vi "Parse Elements Treewise.vi"(4 "VI Data in":T1[](array[typedef]), 5 "XPath Get Attribute":T5[](array[typedef]), 6 "Parents":string[](array[string]), 7 "XPath Node Attribute":T5, 8 "error in":errorcluster, 9 "Attribute":string[](array[string]), 10 "XML File Path":path, 11 "Node in":refnum<k20>) -> (0 "error out":errorcluster, 2 "VI Data out":T1[](array[typedef]), 3 "Node out":refnum<k20>)   [LabVIEW 2020, in "VI Properties Editor.lvlib"]
uses:
  VI Properties Editor.lvlib
  <vilib>/xml/NI_XML.lvlib
  <vilib>/xml/Close Reference(Node).vi
  CTLs/XPath Get Attribute.ctl
  <vilib>/picture/picture.llb/imagedata.ctl
  CTLs/VI Properties.ctl
  CTLs/Control Properties.ctl
  CTLs/VI Data.ctl
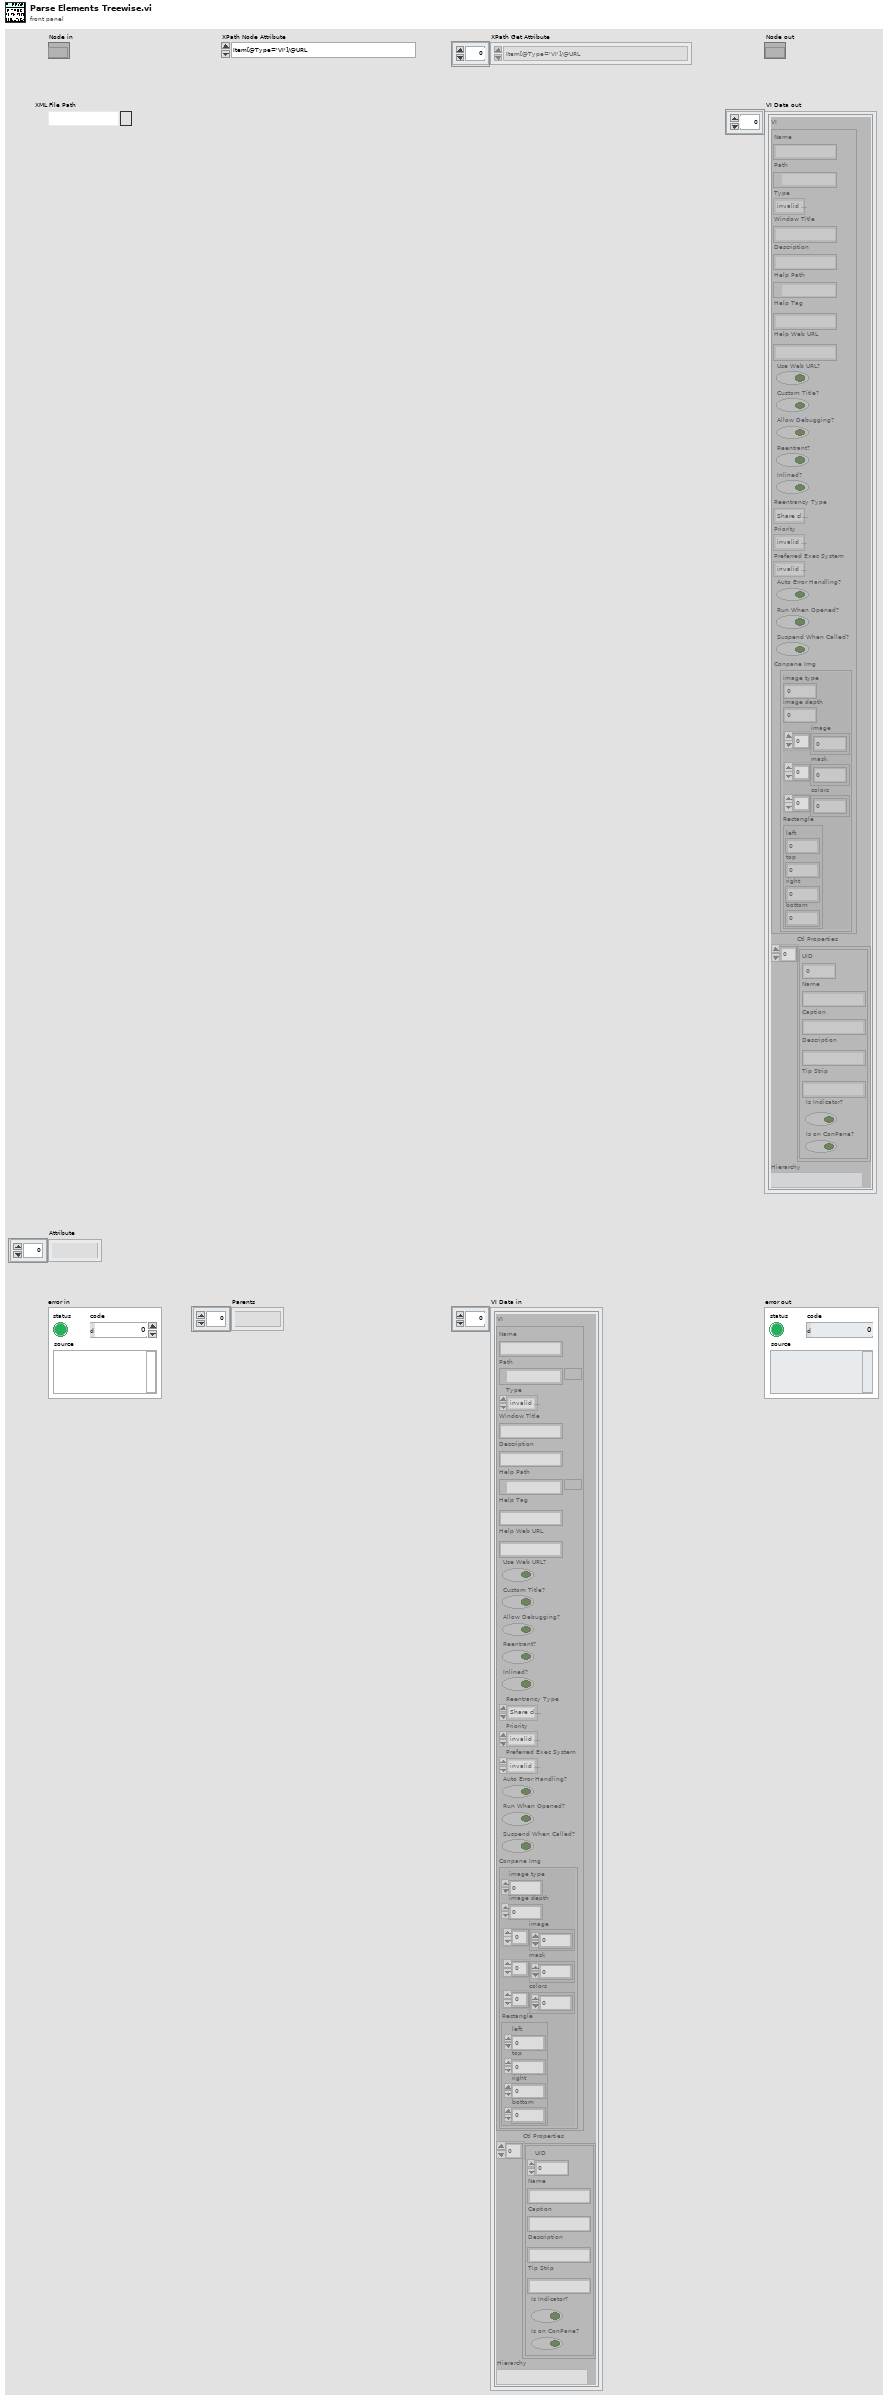
[diagram p1: front panel]
types:
  T1 = typedef "VI Properties Editor.lvlib/VI Data.ctl" = cluster{"VI":T2, "Ctl Properties":T4[], "Hierarchy":string}
  T2 = typedef "VI Properties Editor.lvlib/VI Properties.ctl" = cluster{"Name":string, "Path":path, "Type":enum32{"invalid VI type", "Standard VI", "Control VI", "Global VI", "Polymorphic VI", "Configuration VI", "SubSystem", "Facade VI", "Method VI", "Statechart Diagram VI"}, "Window Title":string, "Description":string, "Help Path":path, "Help Tag":string, "Help Web URL":string, "Use Web URL?":bool, "Custom Title?":bool, "Allow Debugging?":bool, "Reentrant?":bool, "Inlined?":bool, "Reentrancy Type":enum16{"Share clones between instances", "Preallocate clone for each instance"}, "Priority":enum32{"invalid priority", "background priority", "normal priority", "above normal priority", "high priority", "time critical priority", "subroutine"}, "Preferred Exec System":enum32{"invalid execution system", "user interface", "standard", "instrument i/o", "data acquisition", "other 1", "other 2", "same as caller"}, "Auto Error Handling?":bool, "Run When Opened?":bool, "Suspend When Called?":bool, "Conpane Img":T3}
  T3 = typedef "imagedata.ctl" = cluster{"image type":i32, "image depth":i32, "image":u8[], "mask":u8[], "colors":u32[], "Rectangle":cluster{"left":i16, "top":i16, "right":i16, "bottom":i16}}
  T4 = typedef "VI Properties Editor.lvlib/Control Properties.ctl" = cluster{"UID":i32, "Name":string, "Caption":string, "Description":string, "Tip Strip":string, "Is Indicator?":bool, "Is on ConPane?":bool}
  T5 = typedef "VI Properties Editor.lvlib/XPath Get Attribute.ctl" = enum16{"Item[@Type='VI']/@URL", "Item[@Type='LVClass']/@URL", "Item[@Type='Library']/@URL", "Item[@Type='Folder' and not (@URL)]/@Name", "@Name"}
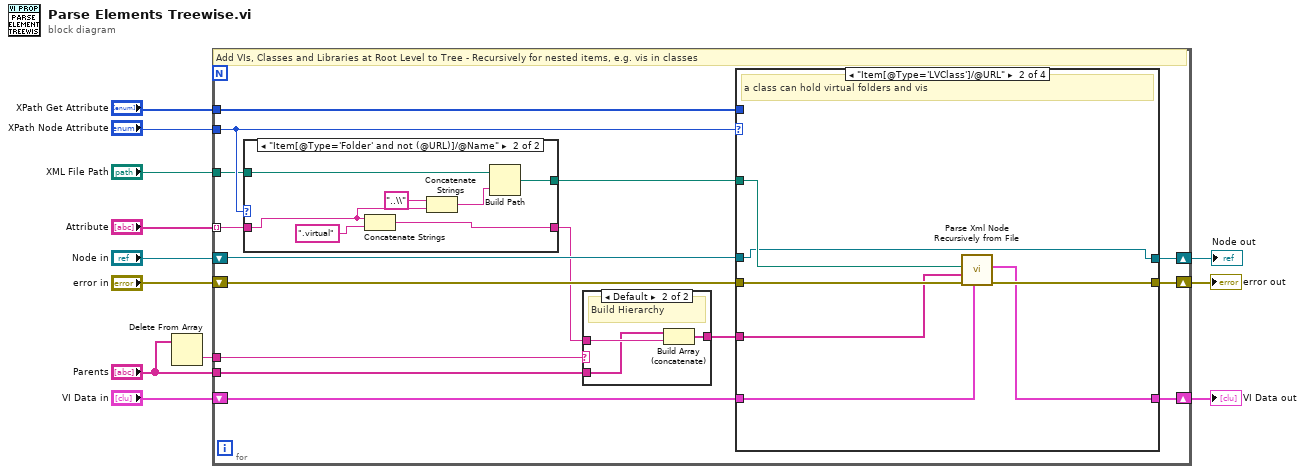
[diagram p0: block diagram]
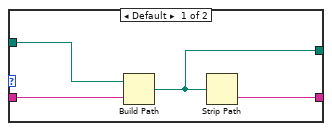
[diagram p2: hidden frame]
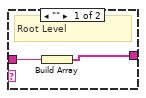
[diagram p3: hidden frame]
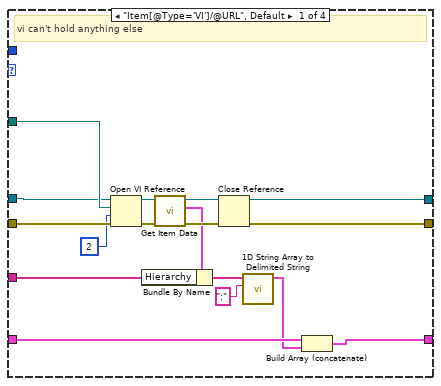
[diagram p4: hidden frame]
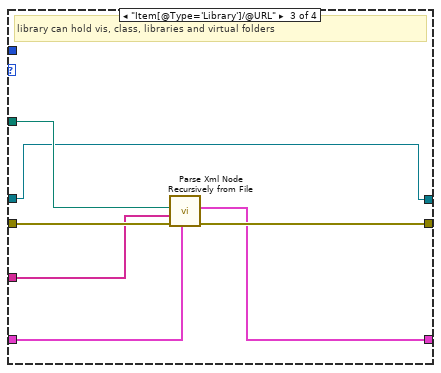
[diagram p5: hidden frame]
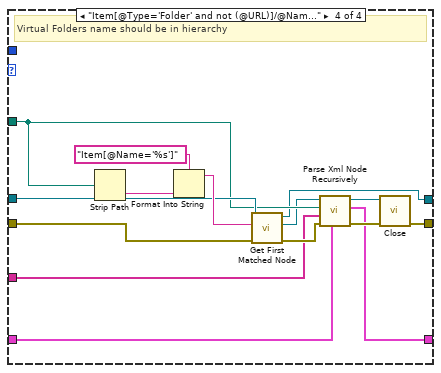
[diagram p6: hidden frame]
diagram:
  n1 = Delete From Array(array="Parents") -> (deleted portion=w2:string)  [unwired: 2 in, 1 out]
  n2 = for {
    shift-right: [w27] -> w5
    shift-left: "error in" -> [w20]
    tunnel: "XPath Node Attribute" -> [w18]
    tunnel: "XML File Path" -> [w15]
    tunnel: "Attribute" -> [w16] mode=indexing
    tunnel: "Parents" -> [w21]
    shift-right: [w24] -> w8
    shift-left: "VI Data in" -> [w23]
    tunnel: "XPath Get Attribute" -> [w25]
    tunnel: w2 -> [w22]
    shift-right: [w13] -> w1
    shift-left: "Node in" -> [w19]
    # "Add VIs, Classes and Libraries at Root Level to Tree - Recursively for nested items, e.g. vis in classes"
    n3 = case shown="\"Item[@Type='Folder' and not (@URL)]/@Name\"" w18 {
      tunnel: w16 -> [w30 w36]
      tunnel: [w29 w37] -> w17
      tunnel: w15 -> [w31 w34]
      tunnel: [w28 w32] -> w14
      frame Default {
        n4 = Build Path(base path=w31, name or relative path=w30) -> (appended path=w28:path)
        n5 = Strip Path(path=w28) -> (name=w29:string)  [unwired: 1 out]
      }
      frame "Item[@Type='Folder' and not (@URL)]/@Name" {
        # "Virtual F."
        n6 = Concatenate Strings(w36, ".virtual" ("string")) -> (w37:string)
        n7 = Concatenate Strings("..\\" ("string"), w36) -> (w33:string)
        n8 = Build Path(base path=w34, name or relative path=w33) -> (appended path=w32:path)
      }
    }
    n9 = case shown="Default" w22 {
      tunnel: w17 -> [w40 w43]
      tunnel: [w39 w42] -> w26
      tunnel: w21 -> [_ w41]
      frame "" {
        # "Root Level"
        n10 = Build Array(w40) -> (w39:string[])
      }
      frame Default {
        # "Build Hierarchy"
        n11 = Build Array (concatenate)(w41, w43) -> (w42:string[])
      }
    }
    n12 = case shown="\"Item[@Type='LVClass']/@URL\"" w18 {
      tunnel: [w55 w66 w72 w87] -> w27
      tunnel: w20 -> [w58 w65 w73 w83]
      tunnel: w14 -> [w45 w64 w71 w81]
      tunnel: w26 -> [w51 w63 w70 w74]
      tunnel: w25 -> [_ _ _ _]
      tunnel: [w46 w61 w68 w77] -> w24
      tunnel: w23 -> [w50 w62 w69 w79]
      tunnel: w19 -> [w44 w60 w67 w84]
      tunnel: [w44 w60 w67 w75] -> w13
      frame "Item[@Type='VI']/@URL", Default {
        # "vi can't hold anything else"
        n13 = Open VI Reference(vi path=w45, options=2, error in (no error)=w58) -> (vi reference=w56:refnum<vi>, error out=w57:errorcluster)  [unwired: 3 in]
        n14 = call "Get Item Data.vi"("error in (no error)"=w57, "VI Ref"=w56) -> ("error out"=w59:errorcluster, "VI Data"=w49:T1, "VI Ref out"=w54:refnum<vi>)  [unwired: 7 in]
        n15 = Close Reference(reference=w54, error in (no error)=w59) -> (error out=w55:errorcluster)
        n16 = call <vilib>:"1D String Array to Delimited String.vi"("delimiter"=":", "string array"=w51) -> ("delimited string"=w47:string)  [unwired: 9 in]
        n17 = Bundle By Name(cluster=w49, "Hierarchy"=w47) -> (w48:T1)
        n18 = Build Array (concatenate)(w50, w48) -> (w46:T1[])
      }
      frame "Item[@Type='LVClass']/@URL" {
        # "a class can hold virtual folders and vis"
        n19 = call "Parse Xml Node Recursively from File.vi"("VI Data"=w62, "error in"=w65, "Parents"=w63, "Path to XML document"=w64) -> ("error out"=w66:errorcluster, "VI Data out"=w61:T1[])  [unwired: 6 in]
      }
      frame "Item[@Type='Library']/@URL" {
        # "library can hold vis, class, libraries and virtual folders"
        n20 = call "Parse Xml Node Recursively from File.vi"("VI Data"=w69, "error in"=w73, "Parents"=w70, "Path to XML document"=w71) -> ("error out"=w72:errorcluster, "VI Data out"=w68:T1[])  [unwired: 6 in]
      }
      frame "Item[@Type='Folder' and not (@URL)]/@Name" {
        # "Virtual Folders name should be in hierarchy"
        n21 = Strip Path(path=w81) -> (name=w80:string)  [unwired: 1 out]
        n22 = Format Into String(format string="Item[@Name='%s']" ("XPath expression"), w80) -> (resulting string=w85:string)  [unwired: 2 in, 1 out]
        n23 = call <vilib>:"Get First Matched Node.vi"("error in (no error)"=w83, "XPath expression"=w85, "node in"=w84) -> ("error out"=w82:errorcluster, "node result"=w78:refnum<k20>, "node out"=w75:refnum<k20>)  [unwired: 6 in]
        n24 = call "Parse Xml Node Recursively.vi"("VI Data"=w79, "error in"=w82, "Parents"=w74, "XML File Path"=w81, "Node in"=w78) -> ("error out"=w88:errorcluster, "VI Data out"=w77:T1[], "Node out"=w76:refnum<k20>)  [unwired: 4 in]
        n25 = call-poly <vilib>:"Close.vi"("error in (no error)"=w88, "node"=w76) -> ("error out"=w87:errorcluster)  [unwired: 7 in]
      }
    }
  }
  "VI Data out" <- w8
  "error out" <- w5
  "Node out" <- w1
